vi "Get ID from JSON.vi"(11 "message json":string) -> (3 "Data out":i32)   [LabVIEW 2025, in "MCP Server.lvlib"]
uses:
  MCP Server.lvlib
  c608c32f-0981-4f1b-93d0-fc5e6564b6e5.vi
  <vilib>/JDP Science/JSONtext/Next JSON Value.vi
  <vilib>/JDP Science/JSONtext/String Subset.vi
  <vilib>/JDP Science/JSONtext/Parsing/Advance past next JSON Value (inlined COPY).vi
  <vilib>/JDP Science/JSONtext/Parsing/Advance past whitespace.vi
  <vilib>/JDP Science/JSONtext/Parsing/Advance past String.vi
  <vilib>/JDP Science/JSONtext/Parsing/Advance past Number.vi
  <vilib>/JDP Science/JSONtext/Parsing/Advance past Line Ending.vi
  <vilib>/JDP Science/JSONtext/Parsing/Parse Full Path or Item Name.vi
  <vilib>/JDP Science/JSONtext/Parsing/Advance past Array.vi
  <vilib>/JDP Science/JSONtext/Parsing/Advance past Object.vi
  <vilib>/JDP Science/JSONtext/support/Error Cluster From Code.vi
  <vilib>/JDP Science/JSONtext/Offset/Find Item Locations by Path.vi
  <vilib>/JDP Science/JSONtext/JSON text to Variant.vi
  <vilib>/JDP Science/JSONtext/LVClass Serializer/JSONtext LVClass Serializer.lvclass
  <vilib>/JDP Science/JSONtext/JSONtext.lvlib
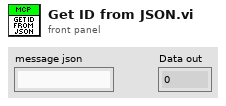
[diagram p1: front panel]
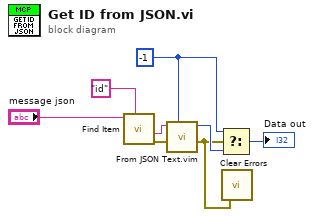
[diagram p0: block diagram]
diagram:
  w2 = -1
  n1 = call <vilib>:"Find Item.vi"("$Path or Item Name"="id", "JSON"="message json") -> ("error out"=w4:errorcluster, "<JSON>"=w6:string)  [unwired: 6 in, 2 out]
  n2 = call "From JSON Text.vim"("Data Type and Default Value"=w2, "error in (no error)"=w4, "JSON"=w6) -> ("error out"=w1:errorcluster, "Data out"=w8:i32)  [unwired: 7 in]
  n3 = Select(t=w2, s=w1, f=w8) -> (s? t:f=→"Data out":i32)
  n4 = call <vilib>:"Clear Errors.vi"("error in (no error)"=w1) -> ()  [unwired: 5 in, 2 out]
